vi "Выработка условия.vi"(7 "String":string) -> (1 "unsigned byte array":u8[](array[numeric]), 2 "sqrt(x)":dbl, 4 "*(type *) &x 8":sgl, 6 "*(type *) &x 9":sgl, 8 "*(type *) &x 10":sgl, 10 "*(type *) &x 11":sgl, 15 "Boolean":bool)   [LabVIEW 2013]
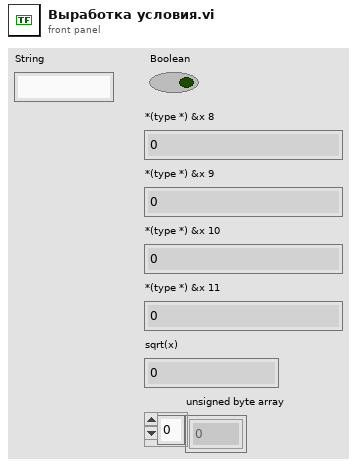
[diagram p1: front panel]
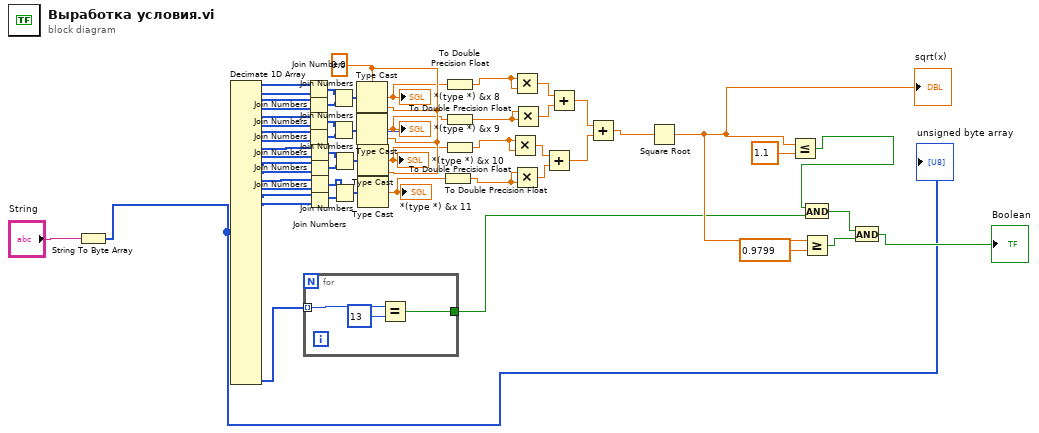
[diagram p0: block diagram]
diagram:
  w54 = sgl 0.0
  n1 = String To Byte Array(string="String") -> (unsigned byte array=w2:u8[])
  "unsigned byte array" <- w2
  n2 = Decimate 1D Array(w2) -> (w15:u8[], w16:u8[], w17:u8[], w18:u8[], w19:u8[], w20:u8[], w21:u8[], w22:u8[], w23:u8[], w24:u8[], w25:u8[], w26:u8[], w27:u8[], w28:u8[], w29:u8[], w30:u8[], w55:u8[])  [unwired: 21 out]
  n3 = Join Numbers(hi=w15, lo=w16) -> ((hi.lo)=w3:u16[])
  n4 = Join Numbers(hi=w17, lo=w18) -> ((hi.lo)=w4:u16[])
  n5 = Join Numbers(hi=w19, lo=w20) -> ((hi.lo)=w5:u16[])
  n6 = Join Numbers(hi=w21, lo=w22) -> ((hi.lo)=w6:u16[])
  n7 = for {
    tunnel: w55 -> [w58] mode=indexing
    tunnel: [w56] -> w48
    n8 = Equal?(x=w58, y=u8 13) -> (x = y?=w56:bool)
  }
  n9 = Join Numbers(hi=w23, lo=w24) -> ((hi.lo)=w8:u16[])
  n10 = Join Numbers(hi=w25, lo=w26) -> ((hi.lo)=w9:u16[])
  n11 = Join Numbers(hi=w27, lo=w28) -> ((hi.lo)=w43:u16[])
  n12 = Join Numbers(hi=w29, lo=w30) -> ((hi.lo)=w44:u16[])
  n13 = Join Numbers(hi=w3, lo=w4) -> ((hi.lo)=w10:u32[])
  n14 = Join Numbers(hi=w5, lo=w6) -> ((hi.lo)=w7:u32[])
  n15 = Join Numbers(hi=w8, lo=w9) -> ((hi.lo)=w13:u32[])
  n16 = Join Numbers(hi=w43, lo=w44) -> ((hi.lo)=w45:u32[])
  n17 = Type Cast(type=w54, x=w10) -> (*(type *) &x=w11:sgl)
  "*(type *) &x 8" <- w11
  n18 = Type Cast(type=w54, x=w7) -> (*(type *) &x=w12:sgl)
  "*(type *) &x 9" <- w12
  n19 = Type Cast(type=w54, x=w13) -> (*(type *) &x=w14:sgl)
  "*(type *) &x 10" <- w14
  n20 = Type Cast(type=w54, x=w45) -> (*(type *) &x=w31:sgl)
  "*(type *) &x 11" <- w31
  n21 = To Double Precision Float(number=w31) -> (double precision float=w35:dbl)
  n22 = To Double Precision Float(number=w11) -> (double precision float=w32:dbl)
  n23 = To Double Precision Float(number=w12) -> (double precision float=w33:dbl)
  n24 = To Double Precision Float(number=w14) -> (double precision float=w34:dbl)
  n25 = Multiply(x=w34, y=w34) -> (x*y=w38:dbl)
  n26 = Multiply(x=w32, y=w32) -> (x*y=w36:dbl)
  n27 = Multiply(x=w35, y=w35) -> (x*y=w39:dbl)
  n28 = Multiply(x=w33, y=w33) -> (x*y=w37:dbl)
  n29 = Add(x=w38, y=w39) -> (x+y=w41:dbl)
  n30 = Add(x=w36, y=w37) -> (x+y=w40:dbl)
  n31 = Add(x=w40, y=w41) -> (x+y=w42:dbl)
  n32 = Square Root(x=w42) -> (sqrt(x)=w51:dbl)
  "sqrt(x)" <- w51
  n33 = Less Or Equal?(x=w51, y=1.1) -> (x <= y?=w47:bool)
  n34 = And(x=w47, y=w48) -> (x .and. y?=w49:bool)
  n35 = Greater Or Equal?(x=w51, y=0.9799) -> (x >= y?=w50:bool)
  n36 = And(x=w49, y=w50) -> (x .and. y?=→"Boolean":bool)
